vi "LJUD U3RAW ConfigIO.vi"(1 "DAC1Enable":u8, 2 "TimerCounterConfig":u8, 4 "EIOAnalog":u8, 6 "FIOAnalog":u8, 7 "Comm Settings":T1={"Open LabJack "=TRUE, "Address"="1", "FirstFound"=TRUE}, 8 "error in (no error)":errorcluster, 10 "WriteMask":u8, 11 "Handle In":i32) -> (0 "error out":errorcluster, 3 "Handle Out":i32)   [LabVIEW 2021]
panel:
  out "Read Array":u8[](array[numeric]) format="%.0x"
  # "If open is false,\nthen a valid\nhandle must be\npassed in."
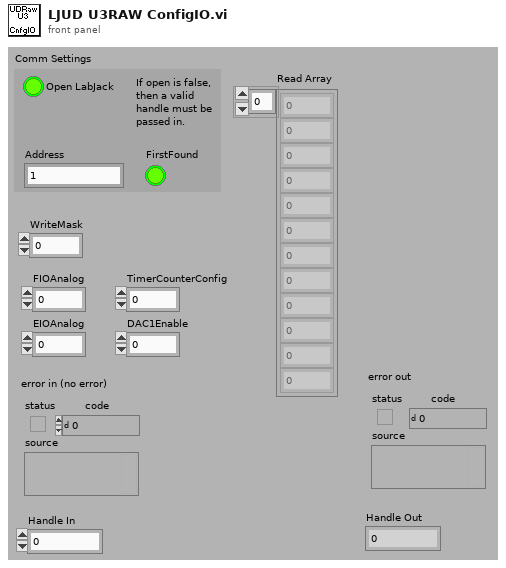
[diagram p1: front panel]
types:
  T1 = cluster{"Open LabJack ":bool, "Address":string, "FirstFound":bool}
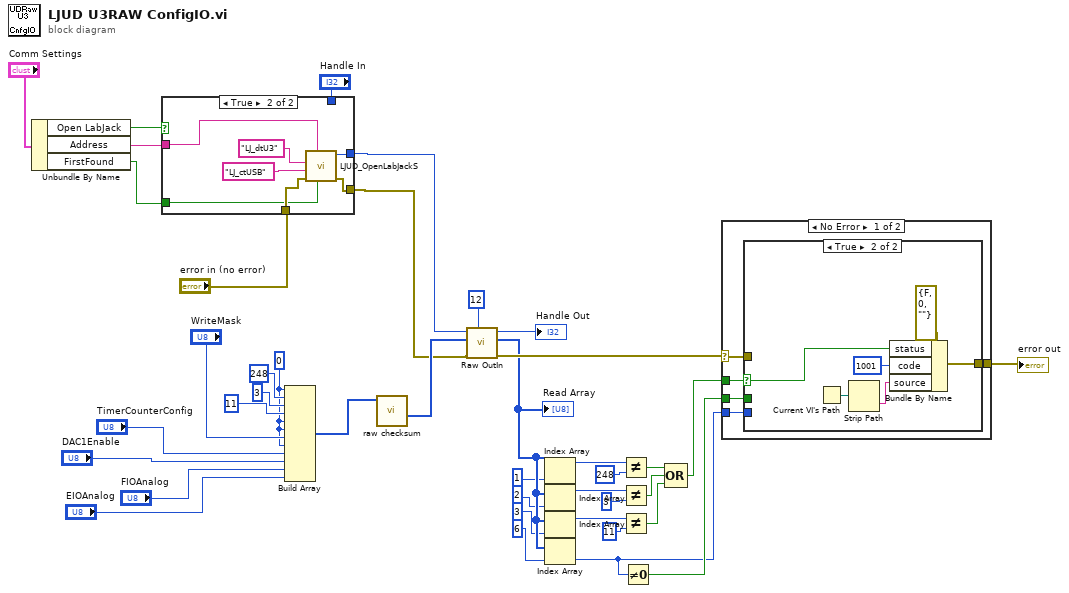
[diagram p0: block diagram]
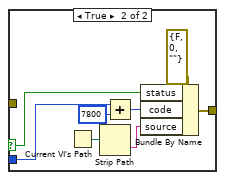
[diagram p3: hidden frame]
diagram:
  w24 = u8 0 ("Input Element")
  n1 = Unbundle By Name("Comm Settings") -> ("Open LabJack"=w27:bool, "Address"=w26:string, "FirstFound"=w25:bool)
  n2 = case shown="True" w27 {
    tunnel: w26 -> [_ w46]
    tunnel: "error in (no error)" -> [w42 w47]
    tunnel: [w42 w48] -> w30
    tunnel: [w41 w49] -> w29
    tunnel: w25 -> [_ w45]
    tunnel: "Handle In" -> [w41 _]
    frame False {
    }
    frame True {
      n3 = call "LJUD_OpenLabJackS.vi"("FirstFound"=w45, "Address"=w46, "error in"=w47, "ConnectionType"="LJ_ctUSB", "DeviceType"="LJ_dtU3") -> ("error out"=w48:errorcluster, "Handle"=w49:i32)  [unwired: 4 in, 1 out]
    }
  }
  n4 = Build Array(w24, u8 248 ("Input Element"), u8 3 ("Input Element"), u8 11 ("Input Element"), w24, w24, "WriteMask", w24, "TimerCounterConfig", "DAC1Enable", "FIOAnalog", "EIOAnalog") -> (w37:u8[])
  n5 = call "raw checksum.vi"("Array"=w37) -> ("Array Output"=w35:u8[])  [unwired: 3 in, 7 out]
  n6 = call "Raw OutIn.vi"("# of bytes to read in"=12 ("# of bytes to read"), "error in"=w30, "Raw Out"=w35, "Handle In"=w29) -> ("error out"=w17:errorcluster, "Raw In"=w9:u8[], "Handle Out"=→"Handle Out":i32)  [unwired: 4 in, 1 out]
  "Read Array" <- w9
  n7 = Index Array(array=w9, index=1 ("Index")) -> (element=w4:u8)
  n8 = Index Array(array=w9, index=2 ("Index")) -> (element=w3:u8)
  n9 = Index Array(array=w9, index=3 ("Index")) -> (element=w2:u8)
  n10 = Index Array(array=w9, index=6 ("Index")) -> (element=w1:u8)
  n11 = Not Equal?(x=w4, y=u8 248 ("Input Element")) -> (x != y?=w20:bool)
  n12 = Not Equal?(x=w3, y=u8 3 ("Input Element")) -> (x != y?=w19:bool)
  n13 = Not Equal?(x=w2, y=u8 11 ("Input Element")) -> (x != y?=w18:bool)
  n14 = Not Equal To 0?(x=w1) -> (x != 0?=w15:bool)
  n15 = Compound Arithmetic op=OR(w20, w19, w18) -> (w16:bool)
  n16 = case shown="No Error" w17 {
    selector: w17 -> [w50 w74]
    tunnel: w16 -> [w54 _]
    tunnel: w15 -> [w53 _]
    tunnel: w1 -> [w52 _]
    tunnel: [w51 w74] -> w14
    frame No Error {
      n17 = case shown="True" w54 {
        selector: w54 -> [_ w68]
        tunnel: w53 -> [w58 _]
        tunnel: w52 -> [w57 _]
        tunnel: [w56 w70] -> w51
        tunnel: w50 -> [w55 _]
        frame False {
          n18 = case shown="False" w58 {
            selector: w58 -> [_ w61]
            tunnel: w57 -> [_ w62]
            tunnel: [w59 w60] -> w56
            tunnel: w55 -> [w59 _]
            frame False {
            }
            frame True {
              n19 = Current VI's Path() -> (path=w65:path)
              n20 = Strip Path(path=w65) -> (name=w64:string)  [unwired: 1 out]
              n21 = Add(x=w62, y=7800) -> (x+y=w66:i32)
              n22 = Bundle By Name(cluster=errorcluster {"status"=FALSE, "code"=0, "source"=""} ("error IO"), "status"=w61, "code"=w66, "source"=w64) -> (w60:errorcluster)
            }
          }
        }
        frame True {
          n23 = Current VI's Path() -> (path=w73:path)
          n24 = Strip Path(path=w73) -> (name=w72:string)  [unwired: 1 out]
          n25 = Bundle By Name(cluster=errorcluster {"status"=FALSE, "code"=0, "source"=""} ("error IO"), "status"=w68, "code"=1001, "source"=w72) -> (w70:errorcluster)
        }
      }
    }
    frame Error {
    }
  }
  "error out" <- w14
